vi "MS Access Reserved Words Set Builder.vi"() -> ()   [LabVIEW 2020, in "ADODB.lvlib"]
uses:
  ADODB.lvlib
  MS Access Reserved Words.ctl
  MS Access Database Engine.lvclass
panel:
  out "Reserved Words":T1
  out "string array":string[](array[string])
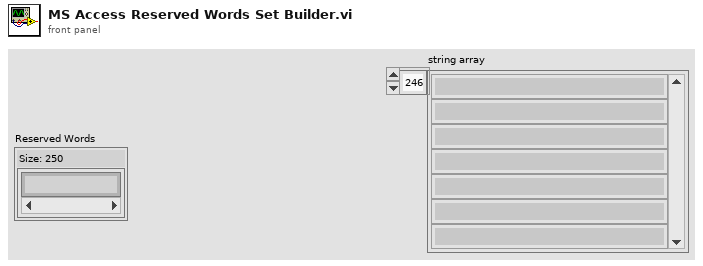
[diagram p1: front panel]
types:
  T1 = typedef "ADODB.lvlib/MS Access Database Engine.lvclass/MS Access Reserved Words.ctl" = set{string}
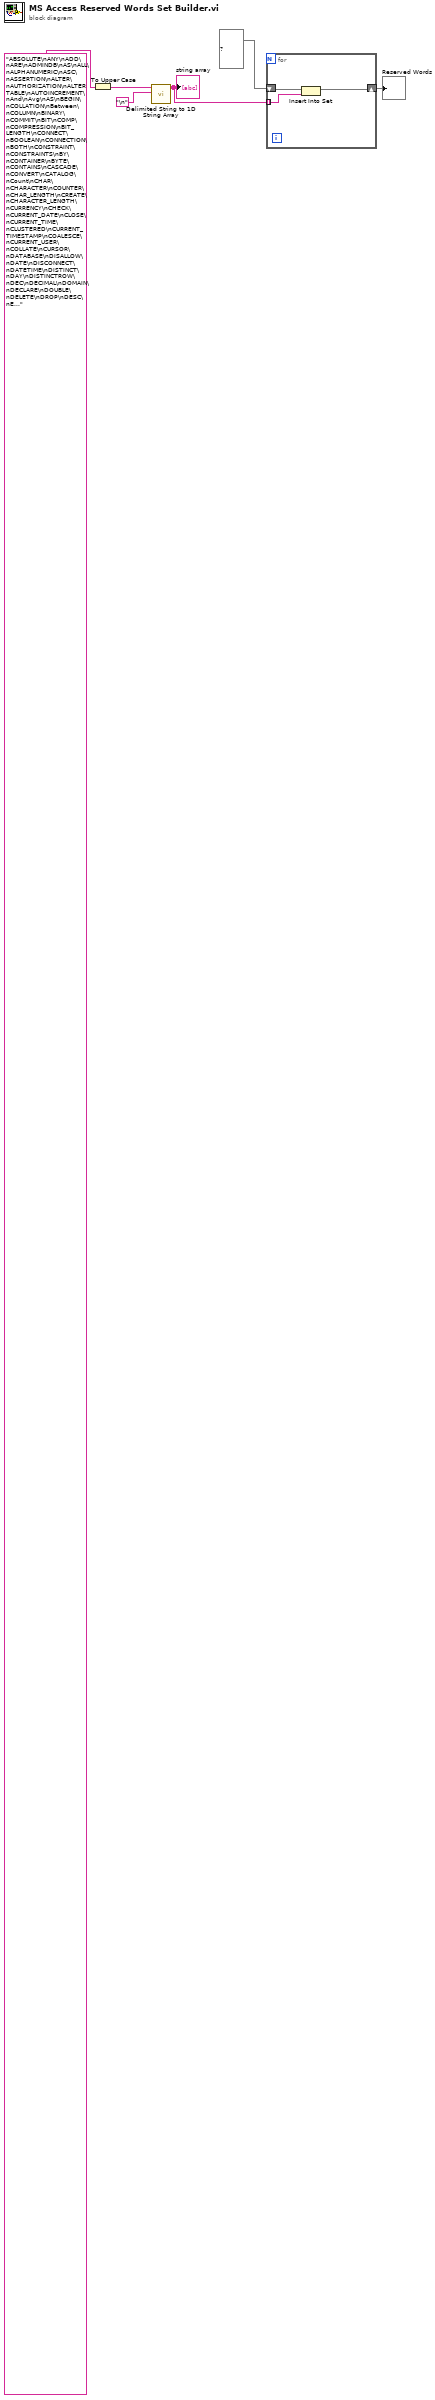
[diagram p0: block diagram]
diagram:
  n1 = To Upper Case(1:"ABSOLUTE\nANY\nADD\nARE\nADMINDB\nAS\nALL\nALPHANUMERIC\nASC\nASSERTION\nALTER\nAUTHORIZATION\nALTER TABLE\nAUTOINCREMENT\nAnd\nAvg\nAS\nBEGIN\nCOLLATION\nBetween\nCOLUMN\nBINARY\nCOMMIT\nBIT\nCOMP\nCOMPRESSION\nBIT_LENGTH\nCONNECT\nBOOLEAN\nCONNECTION\nBOTH\nCONSTRAINT\nCONSTRAINTS\nBY\nCONTAINER\nBYTE\nCONTAINS\nCASCADE\nCONVERT\nCATALOG\nCount\nCHAR\nCHARACTER\nCOUNTER\nCHAR_LENGTH\nCREATE\nCHARACTER_LENGTH\nCURRENCY\nCHECK\nCURRENT_DATE\nCLOSE\nCURRENT_TIME\nCLUSTERED\nCURRENT_TIMESTAMP\nCOALESCE\nCURRENT_USER\nCOLLATE\nCURSOR\nDATABASE\nDISALLOW\nDATE\nDISCONNECT\nDATETIME\nDISTINCT\nDAY\nDISTINCTROW\nDEC\nDECIMAL\nDOMAIN\nDECLARE\nDOUBLE\nDELETE\nDROP\nDESC\nEqv\nFOREIGN\nEXCLUSIVECONNECT\nFROM\nEXEC\nEXECUTE\nFROM\nEXISTS\nGENERAL\nEXTRACT\nGRANT\nFALSE\nGROUP\nFETCH\nGUID\nFIRST\nHAVING\nFLOAT\nFLOAT8\nHOUR\nFLOAT4\nIDENTITY\nINPUT\nIEEEDOUBLE\nINSENSITIVE\nIEEESINGLE\nINSERT\nIGNORE\nINSERT INTO\nIMAGE\nINT\nINTEGER\nINTEGER4\nImp\nINTEGER1\nINTEGER2\nIN\nINTERVAL\nINDEX\nINTO\nINDEXCREATEDB\nIs\nINNER\nISOLATION\nJOIN\nLONGTEXT\nKEY\nLOWER\nLANGUAGE\nMATCH\nLAST\nMax\nLEFT\nMEMO\nLevel\nMin\nLike\nMINUTE\nLOGICAL\nLOGICAL1\nMod\nLONG\nMONEY\nLONGBINARY\nMONTH\nLONGCHAR\nNATIONAL\nOuter\nNCHAR\nOUTPUT\nNONCLUSTERED\nOWNERACCESS\nNot\nPAD\nNTEXT\nPARAMETERS\nNULL\nPARTIAL\nNUMBER\nPASSWORD\nNUMERIC\nPERCENT\nNVARCHAR\nPIVOT\nOCTET_LENGTH\nPOSITION\nOLEOBJECT\nPRECISION\nON\nPREPARE\nOPEN\nPRIMARY\nOPTION\nPRIVILEGES\nOr\nPROC\nPROCEDURE\nORDER\nPUBLIC\nREAL\nSMALLDATETIME\nREFERENCES\nSMALLINT\nRESTRICT\nSMALLMONEY\nREVOKE\nSOME\nRIGHT\nSPACE\nROLLBACK\nSQL\nSCHEMA\nSQLCODE\nSQLERROR\nSQLSTATE\nSECOND\nStDev\nSELECT\nStDevP\nSELECTSCHEMA\nSTRING\nSELECTSECURITY\nSUBSTRING\nSET\nSum\nSHORT\nSYSNAME\nSINGLE\nSYSTEM_USER\nSIZE\nTABLE\nUPDATEOWNER\nTableID\nUPDATESECURITY\nTEMPORARY\nUPPER\nTEXT\nUSAGE\nTIME\nUSER\nTIMESTAMP\nUSING\nTIMEZONE_HOUR\nVALUE\nTIMEZONE_MINUTE\nVALUES\nTINYINT\nVar\nTO\nVARBINARY\nTOP\nVARCHAR\nTRAILING\nVarP\nTRANSACTION\nVARYING\nTRANSFORM\nVIEW\nTRANSLATE\nWHEN\nTRANSLATION\nWHENEVER\nTRIM\nWHERE\nTRUE\nWITH\nUNION\nWORK\nUNIQUE\nXor\nUNIQUEIDENTIFIER\nYEAR\nUNKNOWN\nYESNO\nUPDATE\nZONE\nUPDATEIDENTITY\n") -> (0:w4:string)
  n2 = call <vilib>:"Delimited String to 1D String Array.vi"("delimiter"="\n", "delimited string"=w4) -> ("string array"=w3:string[])  [unwired: 9 in]
  "string array" <- w3
  n3 = for {
    tunnel: w3 -> [w7] mode=indexing
    shift-right: [w8] -> w1
    shift-left: set{string} {} ("set in") -> [w9]
    n4 = Insert Into Set(10:w7, 11:w9) -> (3:w8:set{string})  [unwired: 1 out]
  }
  "Reserved Words" <- w1
